vi "Write Data.vi"(6 "Q":dbl, 8 "error in":errorcluster, 9 "dP":dbl, 10 "P":dbl, 11 "AlicatPData in":refnum<class "AlicatPData.lvclass">) -> (0 "error out":errorcluster, 3 "AlicatPData out":refnum<class "AlicatPData.lvclass">)   [LabVIEW 2014, in "Alicat.lvlib" / "AlicatPData.lvclass"]
uses:
  AlicatPData.lvclass
  AlicatPData.lvclass/AlicatPData.ctl
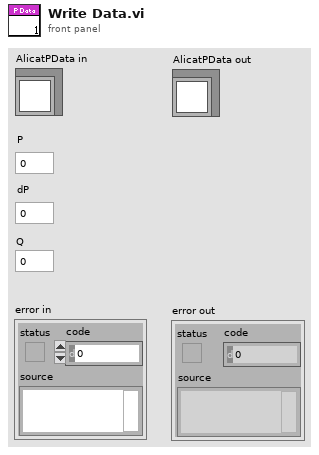
[diagram p1: front panel]
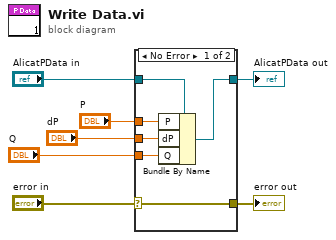
[diagram p0: block diagram]
diagram:
  n1 = case shown="No Error" "error in" {
    selector: "error in" -> [w13 w15]
    tunnel: [w13 w15] -> w6
    tunnel: [w11 w14] -> w4
    tunnel: "AlicatPData in" -> [w12 w14]
    tunnel: "P" -> [w10 _]
    tunnel: "dP" -> [w9 _]
    tunnel: "Q" -> [w8 _]
    frame No Error {
      n2 = Bundle By Name(cluster=w12, "P"=w10, "dP"=w9, "Q"=w8) -> (w11:refnum<class "AlicatPData.lvclass">)
    }
    frame Error {
    }
  }
  "error out" <- w6
  "AlicatPData out" <- w4
